vi "AI-handler.vi"(10 "read buffer in":string) -> (3 "Analog Inputs":T1)   [LabVIEW 2020]
uses:
  controls/analog-input-cluster.ctl
  <vilib>/regexp/Match Regular Expression.xnode
panel:
  out "x <= y?":bool
  out "offset past match":i32
  out "concatenated string":string
  out "match + rest of string":string
  in  "search string/char (-)":string="[+-]"
  out "prototype array":dbl[](array[numeric])
  out "too big cluster":T2
  out "data array":dbl[](array[numeric])
  in  "delimiter (Tab)":string=","
  in  "format string":string
  out "substring":string
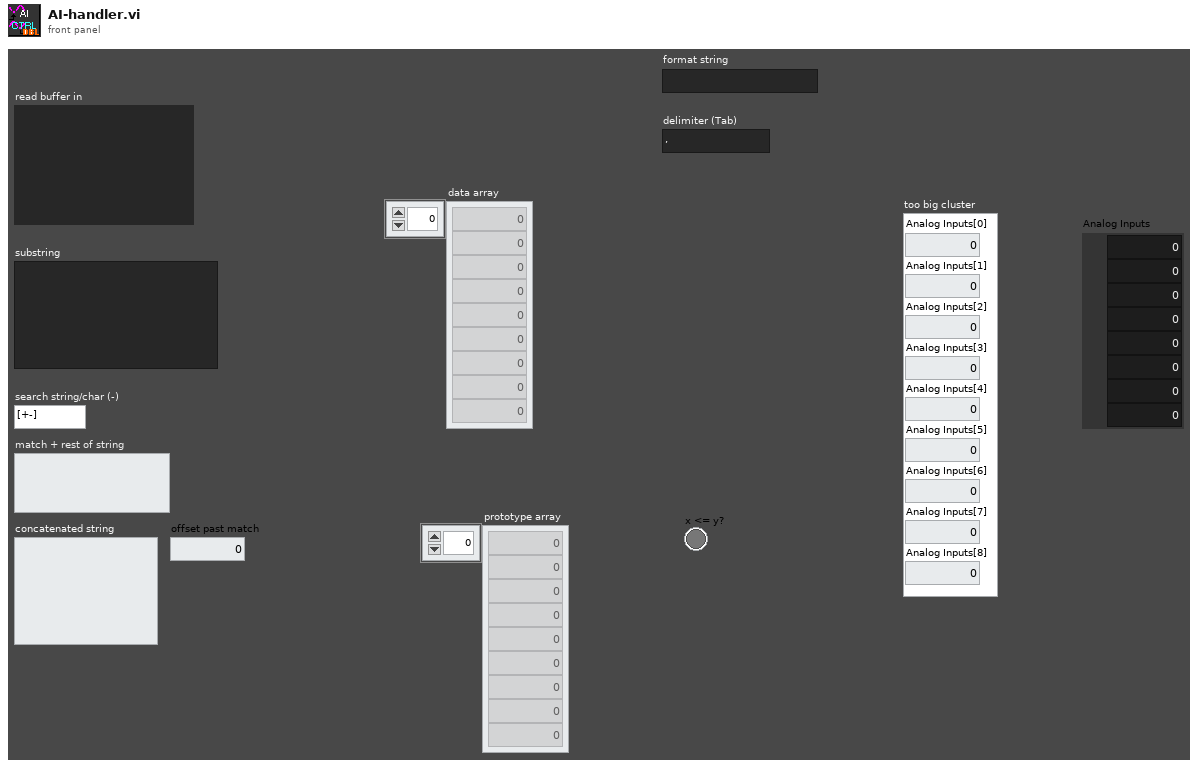
[diagram p1: front panel]
types:
  T1 = typedef "analog-input-cluster.ctl" = cluster{"AI0":dbl, "AI1":dbl, "AI2":dbl, "AI3":dbl, "AI4":dbl, "AI5":dbl, "AI6":dbl, "AI7":dbl}
  T2 = cluster{"Analog Inputs[0]":dbl, "Analog Inputs[1]":dbl, "Analog Inputs[2]":dbl, "Analog Inputs[3]":dbl, "Analog Inputs[4]":dbl, "Analog Inputs[5]":dbl, "Analog Inputs[6]":dbl, "Analog Inputs[7]":dbl, "Analog Inputs[8]":dbl}
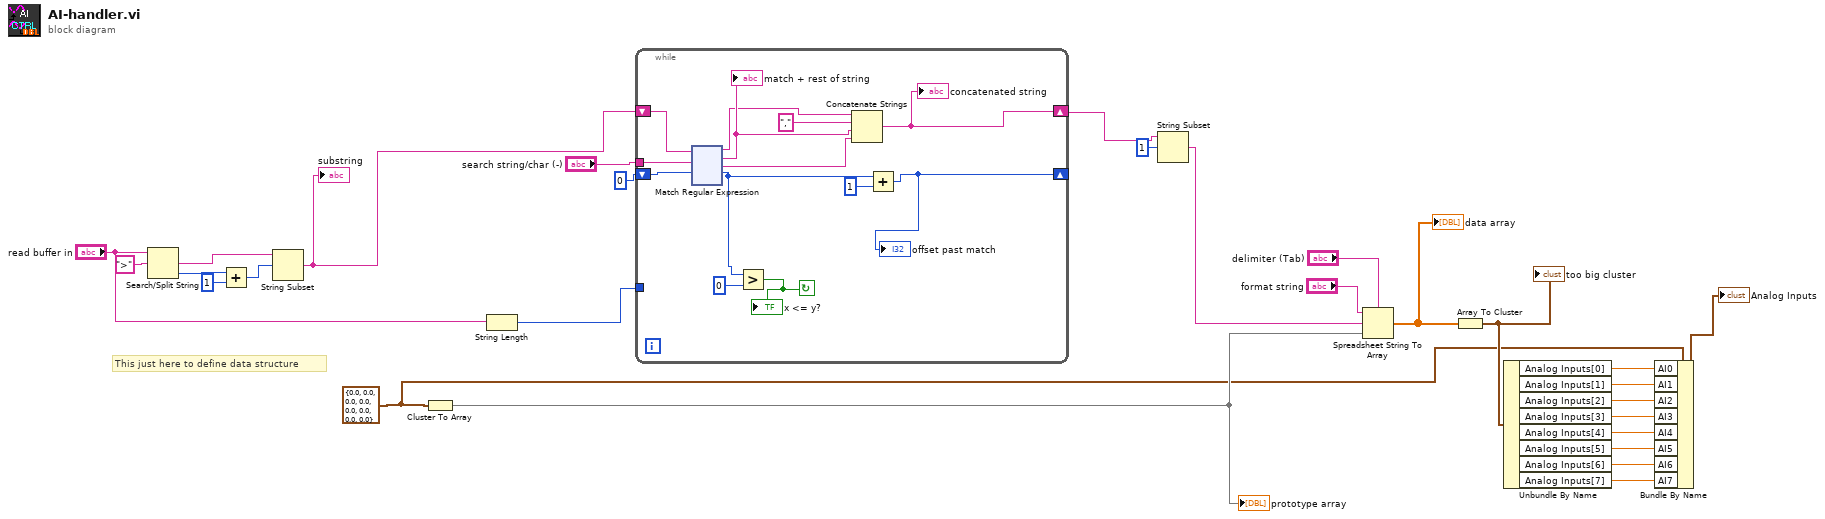
[diagram p0: block diagram]
diagram:
  w13 = T1 {"AI0"=0.0, "AI1"=0.0, "AI2"=0.0, "AI3"=0.0, "AI4"=0.0, "AI5"=0.0, "AI6"=0.0, "AI7"=0.0} ("Analog Inputs")
  # "This just here to define data structure"
  n1 = Search/Split String(string="read buffer in", search string/char (-)=">") -> (match + rest of string=w23:string, offset of match=w24:i32)  [unwired: 1 in, 1 out]
  n2 = Add(x=w24, y=1) -> (x+y=w26:i32)
  n3 = String Subset(string=w23, offset (0)=w26) -> (substring=w15:string)  [unwired: 1 in]
  "substring" <- w15
  n4 = Cluster To Array(cluster=w13) -> (array=w21:dbl[])
  "prototype array" <- w21
  n5 = String Length(string="read buffer in") -> (length=w18:i32)
  n6 = while {
    tunnel: w18 -> [_]
    tunnel: "search string/char (-)" -> [w41]
    shift-right: [w33] -> _
    shift-left: 0 ("offset past match") -> [w36]
    shift-right: [w38] -> w2
    shift-left: w15 -> [w35]
    stop <- w30 continue-if-true
    n7 = xnode ("Match Regular Expression")("input string"=w35, "regular expression"=w41, "offset (0)"=w36) -> ("before match"=w29:string, "whole match"=w40:string, "after match"=w39:string, "offset past match"=w31:i32)  [unwired: 3 in, 1 out]
    "match + rest of string" <- w40
    n8 = Greater?(x=w31, y=0) -> (0:w30:bool)
    "x <= y?" <- w30
    n9 = Concatenate Strings(w29, "," ("string"), w40, w39) -> (w38:string)
    "concatenated string" <- w38
    n10 = Add(x=w31, y=1) -> (x+y=w33:i32)
    "offset past match" <- w33
  }
  n11 = String Subset(string=w2, offset (0)=1) -> (substring=w1:string)  [unwired: 1 in]
  n12 = Spreadsheet String To Array(delimiter (Tab)="delimiter (Tab)", format string="format string", spreadsheet string=w1, array type (2D Dbl)=w21) -> (array=w20:dbl[])
  "data array" <- w20
  n13 = Array To Cluster(array=w20) -> (cluster=w14:T2)
  "too big cluster" <- w14
  n14 = Unbundle By Name(w14) -> ("Analog Inputs[0]"=w12:dbl, "Analog Inputs[1]"=w11:dbl, "Analog Inputs[2]"=w10:dbl, "Analog Inputs[3]"=w9:dbl, "Analog Inputs[4]"=w8:dbl, "Analog Inputs[5]"=w7:dbl, "Analog Inputs[6]"=w6:dbl, "Analog Inputs[7]"=w5:dbl)
  n15 = Bundle By Name(cluster=w13, "AI0"=w12, "AI1"=w11, "AI2"=w10, "AI3"=w9, "AI4"=w8, "AI5"=w7, "AI6"=w6, "AI7"=w5) -> (→"Analog Inputs":T1)
